vi "cleanUpOpenCVIP.vi"() -> (0 "return type":i32)   [LabVIEW 2012]
uses:
  OpenCvGlobals.vi
  <userlib>/OpenCVImProc/CatWalkLabviewDLLd.dll
  <userlib>/OpenCVImProc/CatWalkLabviewDLL.dll
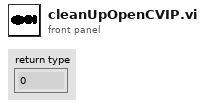
[diagram p1: front panel]
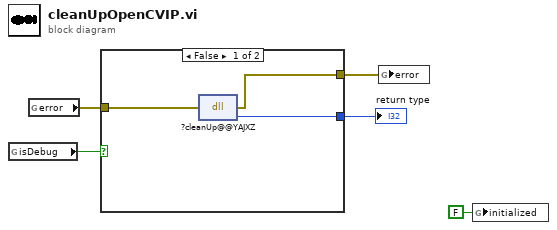
[diagram p0: block diagram]
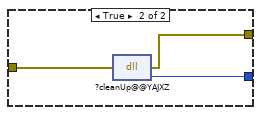
[diagram p2: hidden frame]
diagram:
  n1 = global read "OpenCvGlobals.vi" "isDebug"() -> (w5:bool)
  n2 = global read "OpenCvGlobals.vi" "error"() -> (w2:errorcluster)
  n3 = case shown="False" w5 {
    tunnel: [w6 w11] -> w4
    tunnel: [w7 w9] -> w3
    tunnel: w2 -> [w8 w10]
    frame False {
      n4 = dll-call lib="C:/Program Files (x86)/National Instruments/LabVIEW 2012/user.lib/OpenCVImProc/CatWalkLabviewDLL.dll" fn="?cleanUp@@YAJXZ"(error in=w8) -> (error out=w7:errorcluster, "return type"=w6:i32)  [unwired: 2 in, 1 out]
    }
    frame True {
      n5 = dll-call lib="C:/Program Files (x86)/National Instruments/LabVIEW 2012/user.lib/OpenCVImProc/CatWalkLabviewDLLd.dll" fn="?cleanUp@@YAJXZ"(error in=w10) -> (error out=w9:errorcluster, "return type"=w11:i32)  [unwired: 2 in, 1 out]
    }
  }
  "return type" <- w4
  n6 = global write "OpenCvGlobals.vi" "error"(w3) -> ()
  n7 = global write "OpenCvGlobals.vi" "initialized"(FALSE ("initialized")) -> ()
